vi "stop listening.vi"(8 "error in":errorcluster, 11 "Queue server in":refnum<class "Queue server.lvclass">) -> (0 "error out":errorcluster, 3 "Queue server out":refnum<class "Queue server.lvclass">)   [LabVIEW 2015, in "Queue server.lvclass"]
uses:
  Queue server.lvclass
  Queue Client/opening handshake data.ctl
  message/communicator message.lvclass
  Queue server.lvclass/Queue server.ctl
  message/communicator message.lvclass/communicator message.ctl
  Queue Client/Queue client.lvclass
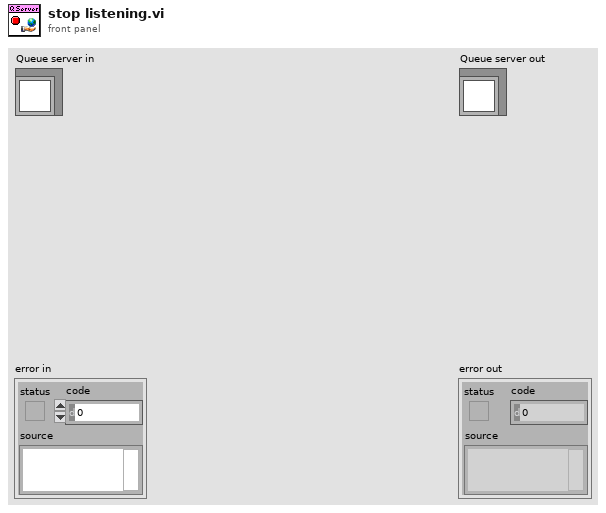
[diagram p1: front panel]
types:
  T1 = typedef "Queue client.lvclass/opening handshake data.ctl" = cluster{"queue":refnum<queue>, "process ID":string}
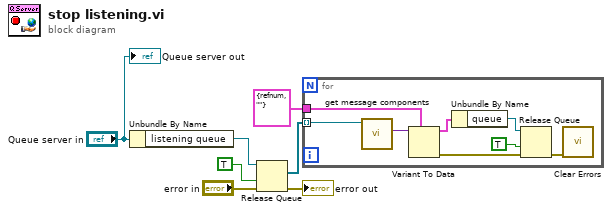
[diagram p0: block diagram]
diagram:
  n1 = Unbundle By Name("Queue server in") -> ("listening queue"=w2:refnum<queue>)
  n2 = Release Queue(queue=w2, force destroy? (F)=TRUE, error in (no error)="error in") -> (remaining elements=w6:refnum<class "communicator message.lvclass">[], error out=→"error out":errorcluster)  [unwired: 1 out]
  n3 = for {
    tunnel: w6 -> [w10] mode=indexing
    tunnel: T1 {"queue"=refnum, "process ID"=""} ("handshake data") -> [w15]
    n4 = call "get message components.vi"("message"=w10) -> ("data"=w9:variant)  [unwired: 9 in, 1 out]
    n5 = Variant To Data(type=w15, Variant=w9) -> (data=w11:T1, error out=w12:errorcluster)  [unwired: 1 in]
    n6 = Unbundle By Name(w11) -> ("queue"=w8:refnum<queue>)
    n7 = Release Queue(queue=w8, force destroy? (F)=TRUE, error in (no error)=w12) -> (error out=w14:errorcluster)  [unwired: 2 out]
    n8 = call <vilib>:"Clear Errors.vi"("error in (no error)"=w14) -> ()  [unwired: 5 in, 2 out]
  }
  "Queue server out" <- "Queue server in"
